vi "Picture_to_IMAQ.vi"(11 "PictureBox":refnum<k24>(container)) -> (3 "IMAQ Image":T1(plugin-control))   [LabVIEW 2016]
uses:
  System.Windows.Forms
  System.Drawing
  <vilib>/wsapi/NI_WebServices.lvlib
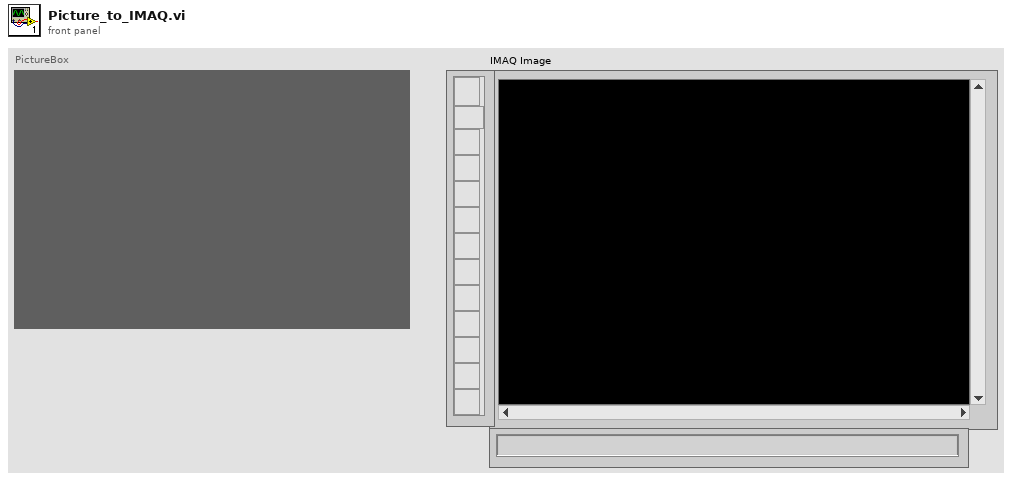
[diagram p1: front panel]
types:
  T1 = typedef "IMAQ Image.ctl" = refnum<image>
  T2 = typedef "Image Type" = u32
  T3 = typedef "imagedata.ctl" = cluster{"image type":i32, "image depth":i32, "image":u8[], "mask":u8[], "colors":u32[], "Rectangle":cluster{"left":i16, "top":i16, "right":i16, "bottom":i16}}
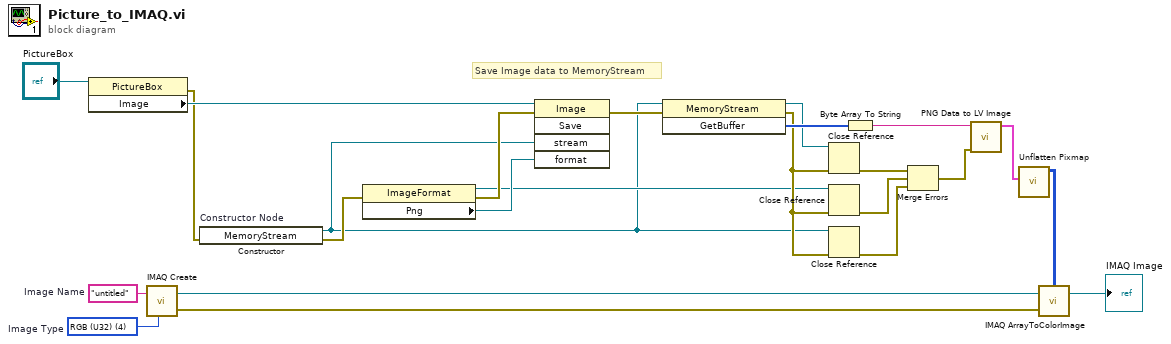
[diagram p0: block diagram]
diagram:
  w23 = "untitled"  # Image Name
  w22 = T2 4 items=["Grayscale (U8)", "Grayscale (I16)", "Grayscale (SGL)", "Complex (CSG)", "RGB (U32)", "HSL (U32)", "RGB (U64)", "Grayscale (U16)"]  # Image Type
  # "Save Image data to MemoryStream"
  n1 = property class="PictureBox"(reference="PictureBox") -> (error out=w10:errorcluster, "Image"=w18:refnum<k24>)  [unwired: 1 in, 1 out]
  n2 = call "IMAQ Create"("Image Name"=w23, "Image Type"=w22) -> ("New Image"=w21:T1, "error out"=w1:errorcluster)  [unwired: 3 in]
  n3 = constructor on="Constructor Node" class="MemoryStream"(error in=w10) -> (reference out=w6:refnum<k24>, error out=w12:errorcluster)  [unwired: 2 in, 1 out]
  n4 = property class="ImageFormat"(error in=w12) -> (reference out=w7:refnum<k24>, error out=w11:errorcluster, "Png"=w14:refnum<k24>)  [unwired: 1 in]
  n5 = invoke class="Image" method="Save"(reference=w18, error in=w11, "stream"=w6, "format"=w14) -> (error out=w13:errorcluster)  [unwired: 1 in, 4 out]
  n6 = invoke class="MemoryStream" method="GetBuffer"(reference=w6, error in=w13) -> (reference out=w9:refnum<k24>, error out=w8:errorcluster, "GetBuffer"=w16:u8[])  [unwired: 1 in]
  n7 = Close Reference(reference=w9, error in (no error)=w8) -> (error out=w5:errorcluster)
  n8 = Close Reference(reference=w7, error in (no error)=w8) -> (error out=w4:errorcluster)
  n9 = Close Reference(reference=w6, error in (no error)=w8) -> (error out=w3:errorcluster)
  n10 = Byte Array To String(unsigned byte array=w16) -> (string=w15:string)
  n11 = Merge Errors "Merge Errors"(w5, w4, w3) -> (w2:errorcluster)
  n12 = call <vilib>:"PNG Data to LV Image.vi"("error in (no error)"=w2, "png data"=w15) -> ("image data"=w17:T3)  [unwired: 8 in, 1 out]
  n13 = call <vilib>:"Unflatten Pixmap.vi"("image data"=w17) -> ("24-bit pixmap"=w20:u32[][])  [unwired: 4 in, 6 out]
  n14 = call "IMAQ ArrayToColorImage"("Image Pixels (U32)"=w20, "Image"=w21, "error in (no error)"=w1) -> ("Image Out"=→"IMAQ Image":T1)  [unwired: 2 in, 1 out]
